vi "RunTimeButtonUI.vi"() -> ()   [LabVIEW 2015, in "RunTimeButton.lvclass"]
uses:
  RunTimeButton.lvclass
  <vilib>/NI/Configuration Framework/Node/NodeRef.ctl
  <vilib>/NI/Configuration Framework/Node/NISE_CEF_Node.lvclass
  <vilib>/NI/AMC/Message Queue.ctl
  <vilib>/NI/AMC/Message.ctl
  <vilib>/NI/Tools/Keyed Array/KeyedArray.ctl
  <vilib>/NI/Configuration Framework/Node/UserEventRef.ctl
  <vilib>/NI/Configuration Framework/Controls/EventCluster.ctl
  RunTimeButton.lvclass/RunTimeButton.ctl
  Read Button Properties.vi
  Write Button Properties.vi
  <vilib>/NI/AMC/Create Single Message.vi
  <vilib>/NI/AMC/Update Message Routing Info.vi
  <vilib>/NI/AMC/Send Message.vi
  <vilib>/NI/AMC/AMC.lvlib
  Configuration Tool.lvlib
  <vilib>/NI/Tools/Keyed Array/Tools_KeyedArray.lvlib
  <vilib>/NI/Configuration Framework/NISE_CEF_TreeControl.lvlib
panel:
  in  "Documentation":string
  in  "Button Type":T1(ring)
  in  "Tip Strip":string
  in  "Caption":string
  in  "Button Text":string
  in  "Dependency Behavior":enum16{"Static", "Dynamic"}(ring)
  in  "Host Path to Dependency File":path
  in  "Host Path to Glyph":path
  in  "Referenced GUID":string="9b525fa0-4d4a-4ec1-902b-bfeef88ebbcc"
  in  "ID":string
  in  "user event":T2
  in  "main queue":T3
  in  "node ref":T4
  # "General Settings"
  # "Dependency File Settings"
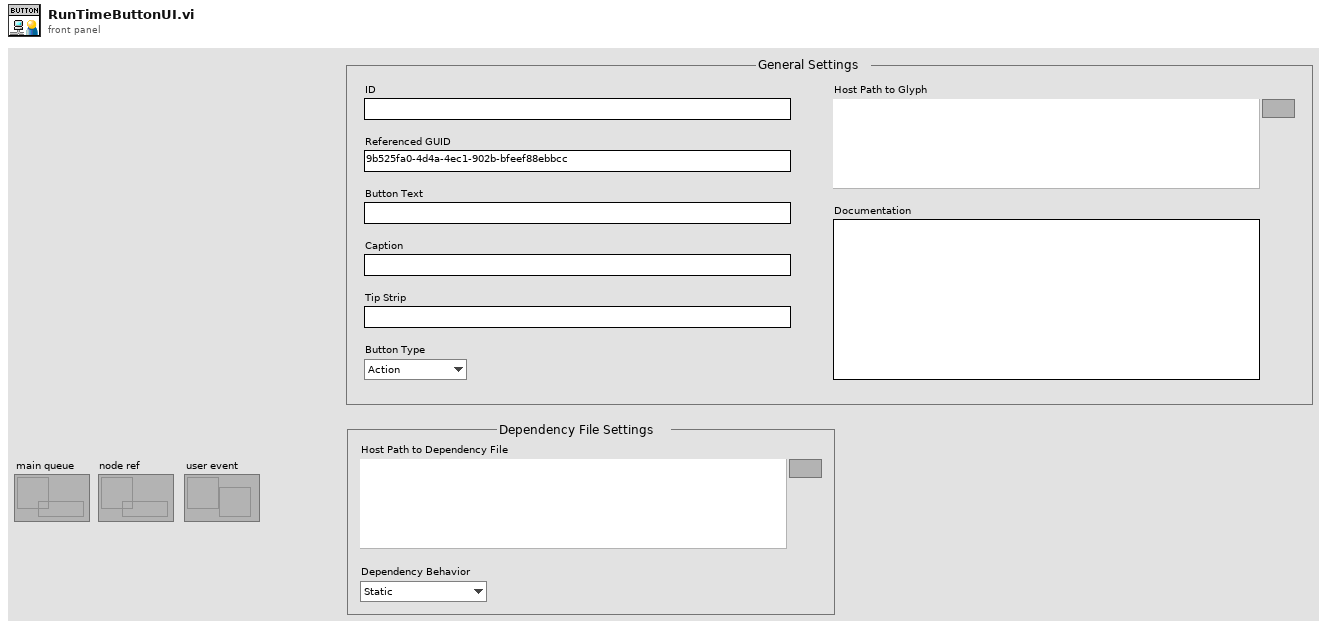
[diagram p1: front panel]
types:
  T1 = enum16{"Action", "Dialog", "Page", "Notification", "Separator"}
  T2 = typedef "NISE_CEF_Node.lvclass/UserEventRef.ctl" = refnum<user-event>
  T3 = typedef "AMC.lvlib/Message Queue.ctl" = refnum<queue>
  T4 = typedef "NISE_CEF_Node.lvclass/NodeRef.ctl" = refnum<data-value>
  T5 = typedef "ButtonLists Properties.ctl" = cluster{"ID":string, "Glyph":T6, "Button Type":T7, "Referenced GUID":string, "Button Text":string, "Caption":string, "Tip Strip":string, "Documentation":string, "Dependency":T8}
  T6 = typedef "Path Cluster.ctl" = cluster{"Path":path, "Path Type":enum16{"Absolute", "To Base", "To Common Doc Dir", "To Application Data Dir"}}
  T7 = typedef "Button Type.ctl" = enum16{"Action", "Dialog", "Page", "Notification", "Separator"}
  T8 = typedef "Dependency three item small.ctl" = cluster{"File Path Control":path, "Path Type":enum16{"Absolute", "To Base", "To Common Doc Dir", "To Application Data Dir"}, "Behavior":enum16{"Static", "Dynamic"}}
  T9 = enum16{"Absolute", "To Base", "To Common Doc Dir", "To Application Data Dir"}
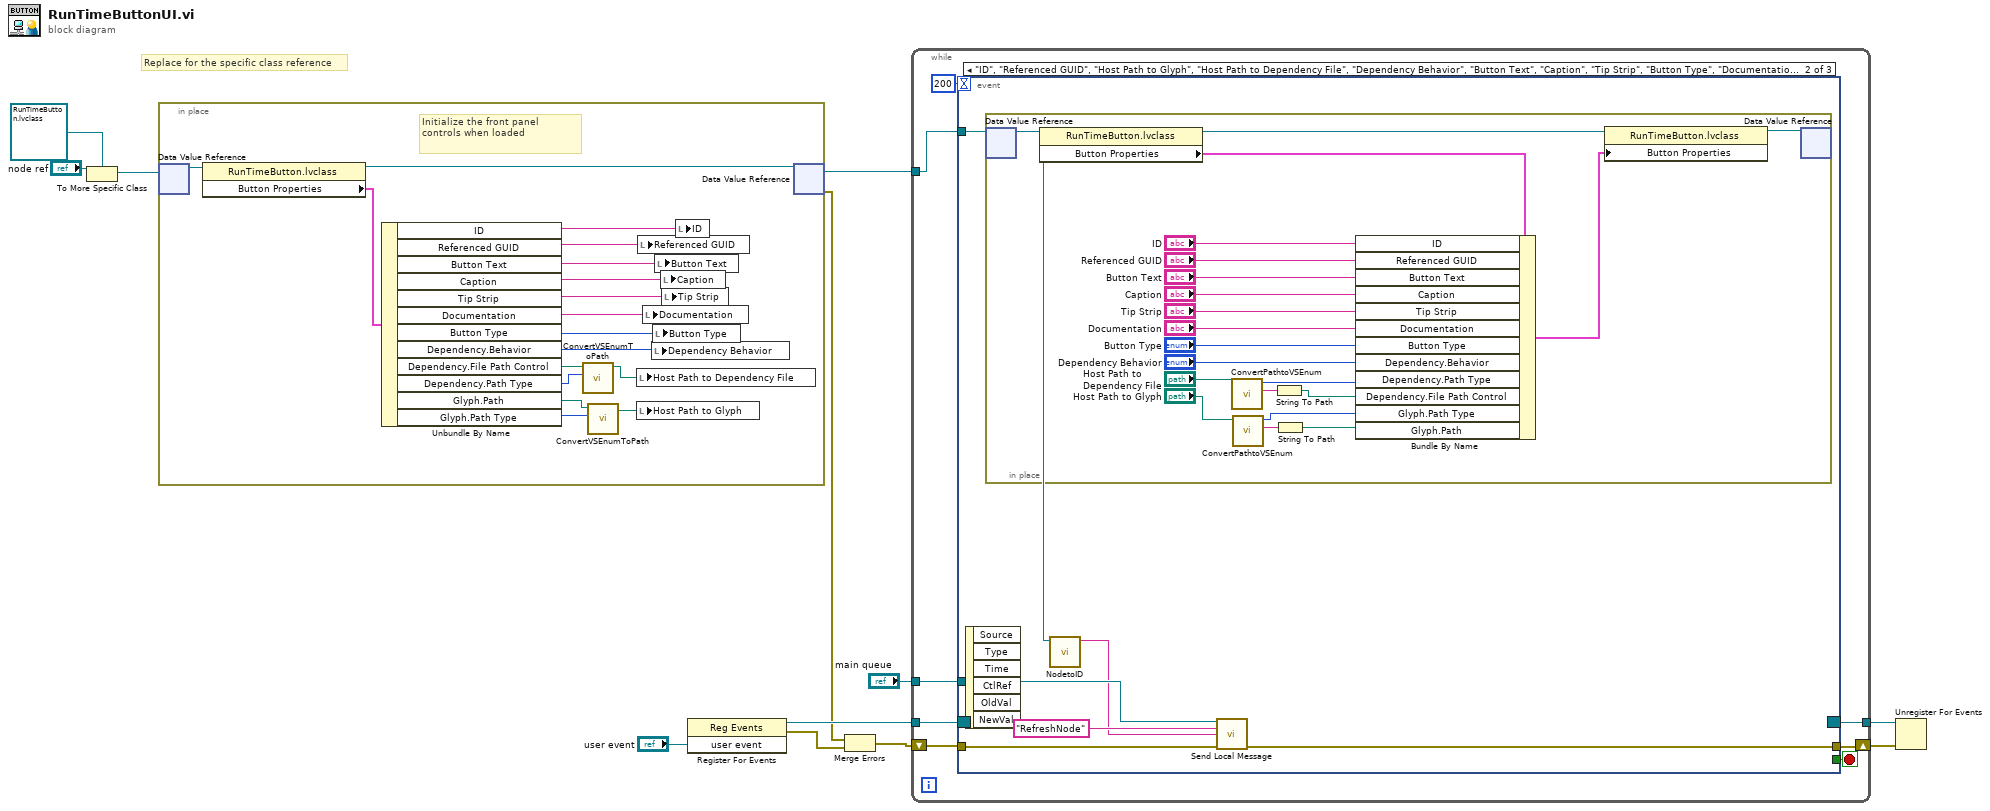
[diagram p0: block diagram]
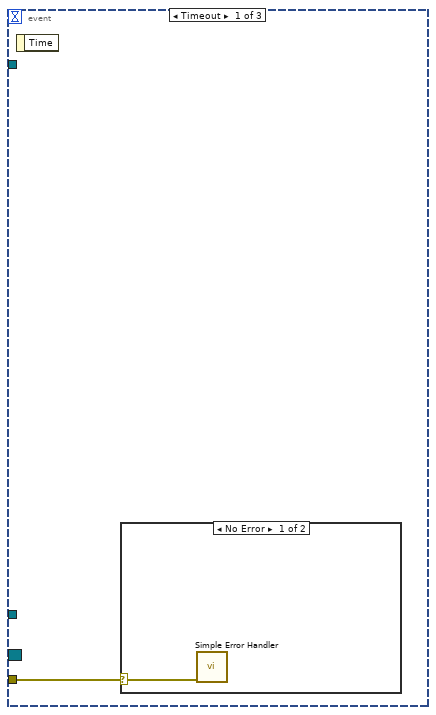
[diagram p2: hidden frame]
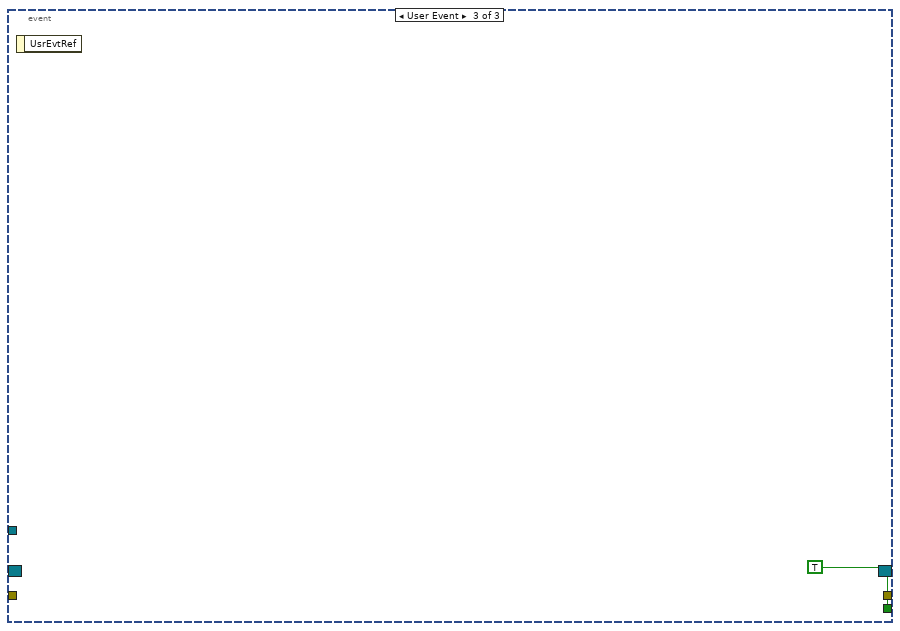
[diagram p4: hidden frame]
diagram:
  # "Replace for the specific class reference"
  n1 = To More Specific Class(target class=refnum<data-value> refnum ("data value reference"), reference="node ref") -> (specific class reference=w5:refnum<data-value>)  [unwired: 1 in, 1 out]
  n2 = in-place {
    # "Initialize the front panel controls when loaded"
    n3 = in-place-dvr #1(w5) -> (w29:refnum<class "RunTimeButton.lvclass">)  [unwired: 1 out]
    n4 = property class="RunTimeButton.lvclass"(reference=w29) -> (reference out=w28:refnum<class "RunTimeButton.lvclass">, "Button Properties"=w27:T5)  [unwired: 1 in, 1 out]
    n5 = Unbundle By Name(w27) -> ("ID"=w26:string, "Referenced GUID"=w25:string, "Button Text"=w24:string, "Caption"=w23:string, "Tip Strip"=w22:string, "Documentation"=w21:string, "Button Type"=w20:T7, "Dependency.Behavior"=w19:enum16{"Static", "Dynamic"}, "Dependency.File Path Control"=w18:path, "Dependency.Path Type"=w17:T9, "Glyph.Path"=w15:path, "Glyph.Path Type"=w14:T9)
    n6 = call "ConvertVSEnumToPath.vi"("Source.Path Type"=w17, "Path In"=w18) -> ("appended path"=w16:path)  [unwired: 9 in]
    n7 = call "ConvertVSEnumToPath.vi"("Source.Path Type"=w14, "Path In"=w15) -> ("appended path"=w13:path)  [unwired: 9 in]
    n8 = local write "Host Path to Dependency File"(w16) -> ()
    n9 = local write "Host Path to Glyph"(w13) -> ()
    n10 = local write "Referenced GUID"(w25) -> ()
    n11 = local write "Documentation"(w21) -> ()
    n12 = local write "Dependency Behavior"(w19) -> ()
    n13 = local write "Button Type"(w20) -> ()
    n14 = local write "Button Text"(w24) -> ()
    n15 = local write "Caption"(w23) -> ()
    n16 = local write "Tip Strip"(w22) -> ()
    n17 = local write "ID"(w26) -> ()
    n18 = in-place-dvr #1(w28) -> (w12:refnum<data-value>, w2:errorcluster)
  }
  n19 = register-events("user event") -> (reference out=w9:refnum<event-registration>, error out=w3:errorcluster)  [unwired: 2 in]
  n20 = Merge Errors(w2, w3) -> (w1:errorcluster)
  n21 = while {
    tunnel: w12 -> [w37]
    tunnel: "main queue" -> [w36]
    tunnel: w9 -> [w34]
    tunnel: [w33] -> w8
    shift-right: [w31] -> w7
    shift-left: w1 -> [w30]
    stop <- w32 stop-if-true
    n22 = event shown="[1] \"ID\", \"Referenced GUID\", \"Host Path to Glyph\", \"Host Path to Dependency File\", \"Dependency Behavior\", \"Button Text\", \"Caption\", \"Tip Strip\", \"Button Type\", \"Documentation\": Value Change" {
      selector: w34 -> [_ _ _]
      dyn-events: [_ _ _] -> w33
      timeout: 200 -> [_ _ _]
      tunnel: w37 -> [_ w43 _]
      tunnel: w36 -> [_ w44 _]
      tunnel: [_ _ TRUE] -> w32
      tunnel: [_ w41 _] -> w31
      tunnel: w30 -> [w38 w40 _]
      event Timeout {
        n23 = event-data() -> ()  [unwired: 1 in, 1 out]
        n24 = case shown="No Error" w38 {
          selector: w38 -> [w39 _]
          frame No Error {
            n25 = call <vilib>:"Simple Error Handler.vi"("error in (no error)"=w39) -> ()  [unwired: 4 in, 5 out]
          }
          frame Error {
          }
        }
      }
      event "ID", "Referenced GUID", "Host Path to Glyph", "Host Path to Dependency File", "Dependency Behavior", "Button Text", "Caption", "Tip Strip", "Button Type", "Documentation": Value Change {
        n26 = event-data() -> ()  [unwired: 1 in, 6 out]
        n27 = in-place {
          n28 = in-place-dvr #2(w43) -> (w64:refnum<class "RunTimeButton.lvclass">)  [unwired: 1 out]
          n29 = property class="RunTimeButton.lvclass"(reference=w64) -> (reference out=w63:refnum<class "RunTimeButton.lvclass">, "Button Properties"=w62:T5)  [unwired: 1 in, 1 out]
          n30 = call "ConvertPathtoVSEnum.vi"("Path In"="Host Path to Dependency File") -> ("Remaining Path"=w65:string, "VS Enum Out"=w51:T9)  [unwired: 9 in]
          n31 = call "ConvertPathtoVSEnum.vi"("Path In"="Host Path to Glyph") -> ("Remaining Path"=w49:string, "VS Enum Out"=w46:T9)  [unwired: 9 in]
          n32 = String To Path(string=w65) -> (path=w50:path)
          n33 = String To Path(string=w49) -> (path=w47:path)
          n34 = Bundle By Name(cluster=w62, "ID"="ID", "Referenced GUID"="Referenced GUID", "Button Text"="Button Text", "Caption"="Caption", "Tip Strip"="Tip Strip", "Documentation"="Documentation", "Button Type"="Button Type", "Dependency.Behavior"="Dependency Behavior", "Dependency.Path Type"=w51, "Dependency.File Path Control"=w50, "Glyph.Path Type"=w46, "Glyph.Path"=w47) -> (w61:T5)
          n35 = property class="RunTimeButton.lvclass"(reference=w63, "Button Properties"=w61) -> (reference out=w66:refnum<class "RunTimeButton.lvclass">)  [unwired: 1 in, 1 out]
          n36 = in-place-dvr #2(w66) -> ()  [unwired: 2 out]
        }
        n37 = call <vilib>:"NodetoID.vi"("node ref"=w43) -> ("ID"=w42:string)  [unwired: 9 in, 1 out]
        n38 = call <vilib>:"Send Local Message.vi"("message queue in"=w44, "message name"="RefreshNode" ("Message Name"), "message value"=w42, "error in"=w40) -> ("error out"=w41:errorcluster)  [unwired: 9 in, 2 out]
      }
      event User Event {
        n39 = event-data() -> ()  [unwired: 1 in, 1 out]
      }
    }
  }
  n40 = Unregister For Events(event registration refnum=w8, error in=w7) -> ()  [unwired: 1 out]
